vi "Motion Profile Generator-Target Speed-Optimized.vi"(8 "Motion Profile Control Frame Rate":dbl=10.0, 9 "Target Speed":dbl=4.0, 10 "Max Jerk (rotations/sec^2)":dbl=1.0, 11 "Max Acceleration (rotations/sec)":dbl=3.0) -> (3 "velocity rotations/sec":dbl[](array[numeric]))   [LabVIEW 2015]
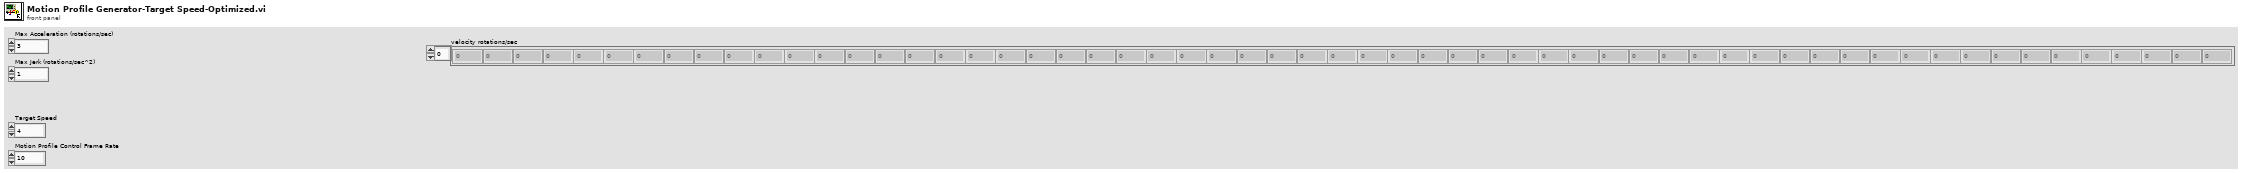
[diagram p1: front panel]
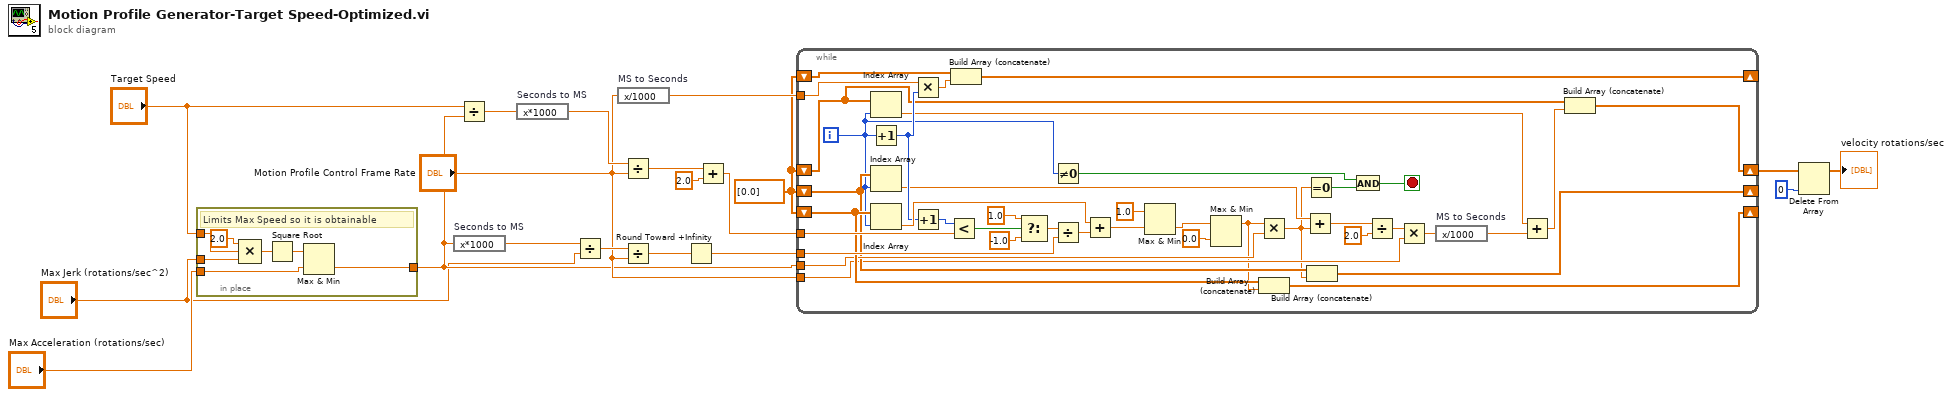
[diagram p0: block diagram]
diagram:
  w8 = dbl[] [0.0]
  n1 = in-place {
    in-place-border: "Max Acceleration (rotations/sec)" -> [w26]
    in-place-border: [w24] -> w6
    in-place-border: "Max Jerk (rotations/sec^2)" -> [w20]
    in-place-border: "Target Speed" -> [w21]
    # "Limits Max Speed so it is obtainable"
    n2 = Compound Arithmetic op=MULTIPLY(2.0 ("x"), w21, w20) -> (w23:dbl)
    n3 = Square Root(x=w23) -> (sqrt(x)=w22:dbl)
    n4 = Max & Min(x=w22, y=w26) -> (min(x,y)=w24:dbl)  [unwired: 1 out]
  }
  n5 = expression code="x*1000" "Seconds to MS"(w6) -> (w18:dbl)
  n6 = Divide(x="Target Speed", y=w6) -> (x/y=w17:dbl)
  n7 = expression code="x*1000" "Seconds to MS"(w17) -> (w16:dbl)
  n8 = Divide(x=w18, y="Max Jerk (rotations/sec^2)") -> (x/y=w12:dbl)
  n9 = expression code="x/1000" "MS to Seconds"("Motion Profile Control Frame Rate") -> (w19:dbl)
  n10 = Divide(x=w16, y="Motion Profile Control Frame Rate") -> (x/y=w15:dbl)
  n11 = Divide(x=w12, y="Motion Profile Control Frame Rate") -> (x/y=w11:dbl)
  n12 = Round Toward +Infinity(x=w11) -> (ceil(x): smallest int >= x=w10:dbl)
  n13 = Add(x=w15, y=2.0) -> (x+y=w13:dbl)
  n14 = while {
    shift-right: [w65] -> _
    shift-left: w8 -> [w66]
    tunnel: w19 -> [w64]
    tunnel: w13 -> [w62]
    shift-right: [w48] -> _
    shift-left: w8 -> [w47]
    tunnel: w10 -> [w54]
    tunnel: w6 -> [w46]
    shift-right: [w45] -> _
    shift-left: w8 -> [w43]
    shift-right: [w44] -> w3
    shift-left: w8 -> [w37]
    tunnel: "Motion Profile Control Frame Rate" -> [w33]
    i -> [w32]
    stop <- w28 stop-if-true
    n15 = Index Array(array=w37, index=w32) -> (element=w36:dbl)
    n16 = Increment(x=w32) -> (x+1=w50:i32)
    n17 = Index Array(array=w43, index=w32) -> (element=w34:dbl)
    n18 = Index Array(array=w47, index=w32) -> (element=w52:dbl)
    n19 = Multiply(x=w64, y=w50) -> (x*y=w63:dbl)
    n20 = Increment(x=w50) -> (x+1=w51:i32)
    n21 = Less?(x=w51, y=w62) -> (x < y?=w58:bool)
    n22 = Build Array (concatenate)(w66, w63) -> (w65:dbl[])
    n23 = Select(t=1.0, s=w58, f=-1.0) -> (s? t:f=w55:dbl)
    n24 = Not Equal To 0?(x=w32) -> (x != 0?=w29:bool)
    n25 = Divide(x=w55, y=w54) -> (x/y=w53:dbl)
    n26 = Add(x=w52, y=w53) -> (x+y=w49:dbl)
    n27 = Max & Min(x=1.0, y=w49) -> (min(x,y)=w60:dbl)  [unwired: 1 out]
    n28 = Max & Min(x=w60, y=0.0) -> (max(x,y)=w27:dbl)  [unwired: 1 out]
    n29 = Multiply(x=w27, y=w46) -> (x*y=w31:dbl)
    n30 = Build Array (concatenate)(w47, w27) -> (w48:dbl[])
    n31 = Add(x=w34, y=w31) -> (x+y=w42:dbl)
    n32 = Equal To 0?(x=w31) -> (x = 0?=w30:bool)
    n33 = Build Array (concatenate)(w43, w31) -> (w45:dbl[])
    n34 = And(x=w29, y=w30) -> (x .and. y?=w28:bool)
    n35 = Divide(x=w42, y=2.0) -> (x/y=w40:dbl)
    n36 = Multiply(x=w40, y=w33) -> (x*y=w39:dbl)
    n37 = expression code="x/1000" "MS to Seconds"(w39) -> (w38:dbl)
    n38 = Add(x=w36, y=w38) -> (x+y=w35:dbl)
    n39 = Build Array (concatenate)(w37, w35) -> (w44:dbl[])
  }
  n40 = Delete From Array(array=w3, index=0) -> (array with subset deleted=→"velocity rotations/sec":dbl[])  [unwired: 1 in, 1 out]
